vi "CPP-BLplotter.vi"(0 "Plot Array":cluster{dbl[], dbl[]}[](array[cluster]) {"?" format="%.2f"; "?" format="%.2f"}, 1 "Job Directory":path) -> (2 "Saved Automatically?":bool, 3 "gnuplotScript":string, 4 "Plot data file":path)   [LabVIEW 2015]
uses:
  gnuplotScriptComponents/BLPlottersubVIs/BLTarget.ctl
  gnuplotScriptComponents/BLPlottersubVIs/Resampler.ctl
  gnuplotScriptComponents/at.ctl
  Results_plotter_Global.vi
panel:
  in  "Tab Control":enum32{"Good Shit", "Targets", "Boring Shit"}(tab)
  in  "NormaliseHeight?":bool
  in  "oneshot":bool=TRUE
  in  "U(h)":dbl min=0.0 step=0.5
  in  "Fit Zmin":dbl=100.0 min=0.0 max=200.0 step=20.0
  in  "autoprint":bool
  out "with d0":cluster{"n":dbl, "d0":dbl, "d0 2":dbl} {"d0 2" format="%#.1e"; "d0" format="%#.1f"; "n" format="%.3f"}
  in  "Fit Zmax":dbl=550.0 min=0.0 max=2000.0 step=50.0
  out "lambda-":dbl format="%_2g"
  out "lambda+":dbl format="%_2g"
  out "lambda(h)":dbl format="%.3g"
  in  "HeightJitter%":dbl min=0.0 max=20.0 step=1.0
  in  "Spectra Folder::":path
  out "Spectrum":cluster{"all rows":dbl[], "all rows":dbl[]}[](graph)
  in  "Stop Button":bool
  in  "Print Button":bool
  out "U,L(U)":cluster{dbl[], dbl[]}[](graph)
  out "TI,Sigma":cluster{dbl[], dbl[]}[](graph)
  in  "MaxFitFreq":dbl
  in  "lambdaSpan(%)":dbl
  in  "integralTweak":dbl=1.0 min=0.8 max=3.0 step=0.01
  out "case":string
  out "No d0":cluster{"n":dbl, "d0":dbl, "d0 2":dbl} {"d0 2" format="%#.1e"; "n" format="%.3f"}
  in  "Spectra?":bool
  in  "Scale":dbl=1.0 min=1.0 max=10000.0 step=50.0
  in  "Zref":dbl=508.0 min=0.0 step=25.0
  in  "BL Scratchpad":T1[](array[typedef]) {"n" min=0.02 max=0.5 step=0.01 format="%.2f"}
  in  "Boundary Layer Targets Folder":path=path "Data plotting/BLplotterExampleProfiles"
  out "BL Targets":T1[](array[typedef]) {"n" min=0.02 max=0.5 step=0.01 format="%.2f"}
  in  "ScaleInTitle?":bool
  in  "OutputType":enum16{"PDF", "PNG-ReportStyle"}(ring)
  out "File Path Control":path
  in  "Resampler":T2
  in  "ResampleToN":i32=12
  in  "ResampleHeights":dbl[](array[numeric])=[25.4, 38.1, 50.8, 76.2, 101.6, 127.0, 152.4, 203.2, 254.0, 304.8, 406.4, 508.0, 609.6, 812.8, 1219.2, 1524.0]
  in  "Use for:":T3(array[ring])=[enum."\nU", enum."\nLambda", enum."\nTI", enum."\nSigma"]
  out "Incoming Titles":string[](array[string])
  in  "Plot Title":u16(ring) items=["Title String Only", "X:Ref:", "Z:Ref:", "Uref::", "X::", "Y::", "Z::", "U/U_{ref}::", "TI(U)::(%)", "\\lambda(U)::(mm)", "\\sigma(U)/U_{ref}::", "U::", "Var(U)::", "tau(U)::", "Spire::", "Trip::", "Rough::", "Addl::", "Date::", "Seconds::", "Comments::", "Run:Messages:", "Reference:Temperature:Used for Corrections", "Atmos:Pressure:Used for Corrections", "Multi Run:Start Time:", "Measuring:Instrument:Type", "Descpn::", "Multi Run:Row:Type", "Raw:Data:Filename", "Original:Results:Filename", "Current:Data:Filename", "Source::", "n:Regular: Z 80.0 - 800.0", "nd:Regular: Z 80.0 - 800.0", "d0:Regular: Z 80.0 - 800.0", "TI:at:200", "TI:at:400", "TI:at:800", "CandidateFor::", "Z-d::", "Trip:Loc:", "Spires:Loc:", "Number of Measurements"]
  out "Final Title":string
  in  "Plot Title Post Block":string
  in  "Plot Title Pre Block":string="Test"
  in  "Show Script Editor?":bool
  in  "OpenLogfile?":bool
  out "spectraLegend":string[](array[string])
  in  "SpecificPlotFolder":string="DescriptiveFolderName"
  # "Fit using values at  measurement Z heights"
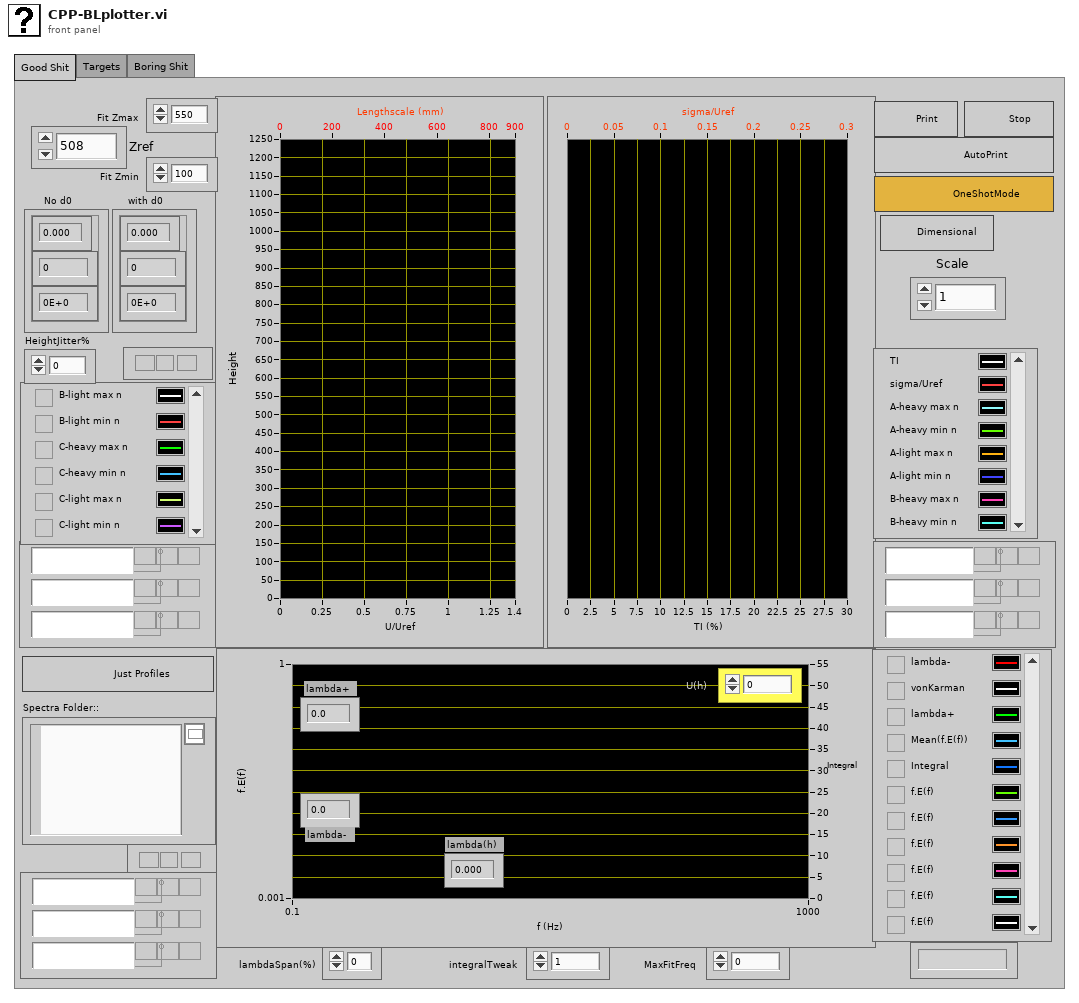
[diagram p1: front panel]
types:
  T1 = typedef "BLTarget.ctl" = cluster{"Code":string, "TI Profile (FS)":dbl[][], "n":dbl}
  T2 = typedef "Resampler.ctl" = enum32{"AsTaken", "Regular", "Prescribed"}
  T3 = enum16{"Don't Use", "\nU", "\nLambda", "\nTI", "\nSigma"}[]
  T4 = typedef "at.ctl" = cluster{"XcoordSys":string, "YcoordSys":string, "Xvalue":dbl, "Yvalue":dbl}
  T5 = typedef "LVRangeTypeDef.ctl" = cluster{"Minimum":dbl, "Maximum":dbl, "Increment":dbl, "Minor Increment":dbl, "Start":dbl}
  T6 = typedef "PowerLaw.ctl" = cluster{"n":dbl, "d0":dbl, "Residual":dbl}
  T7 = cluster{"TI Profile (FS)":dbl[], "Array":dbl[]}[]
  T8 = cluster{"Array":dbl[], "best nonlinear fit":dbl[]}
  T9 = cluster{"Plot.Plot Name":string, "Plot.Plot Color":u32, "Plot.Visible?":bool}
  T10 = typedef "minAndMax.ctl" = cluster{"Min":T11, "Max":T11}
  T11 = typedef "AutoManualNumber.ctl" = cluster{"Auto":bool, "Value":dbl}
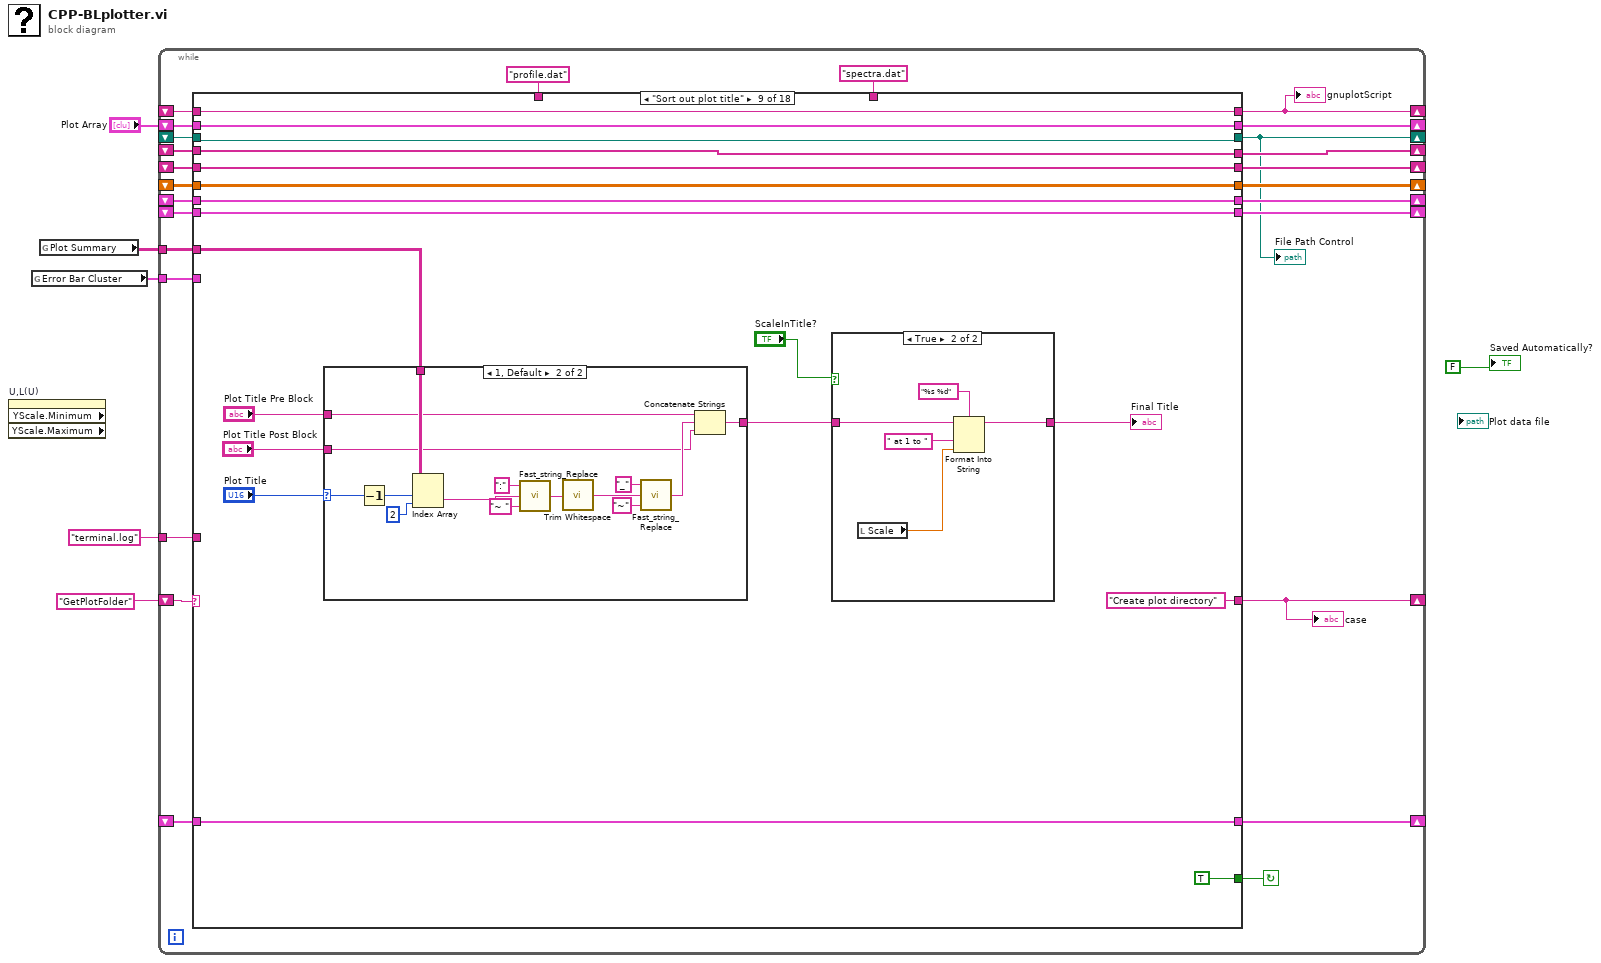
[diagram p0: block diagram]
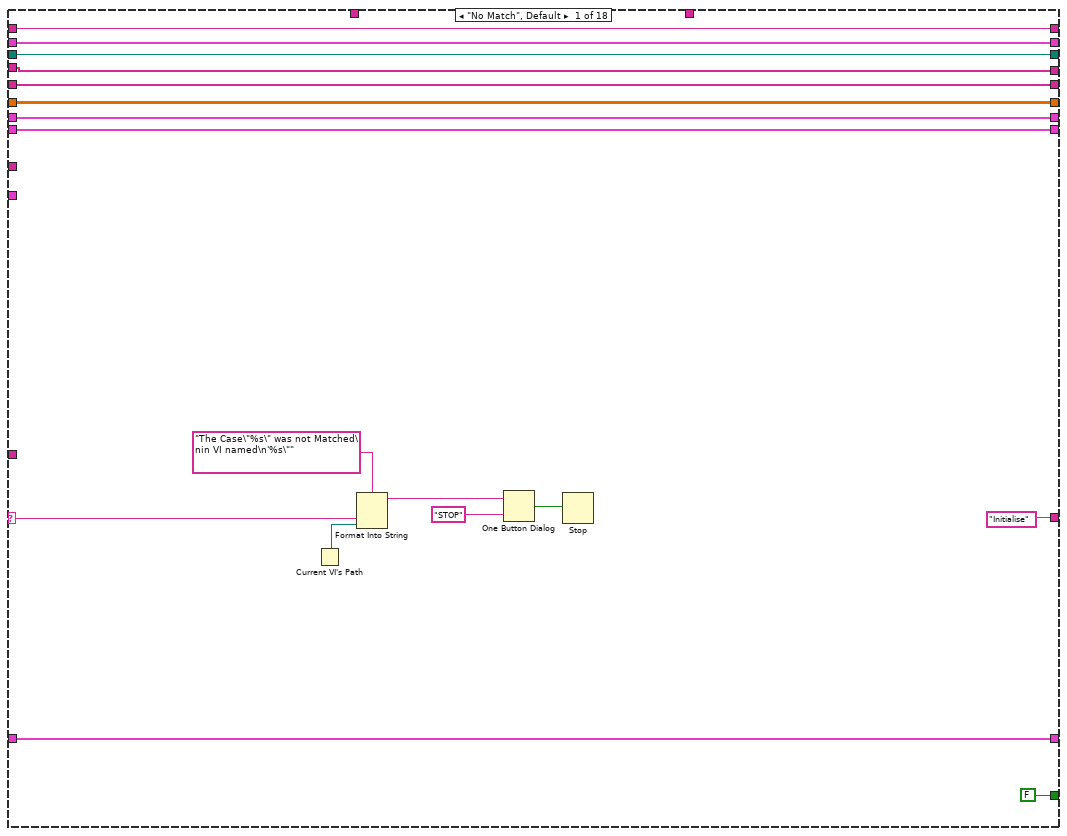
[diagram p2: hidden frame]
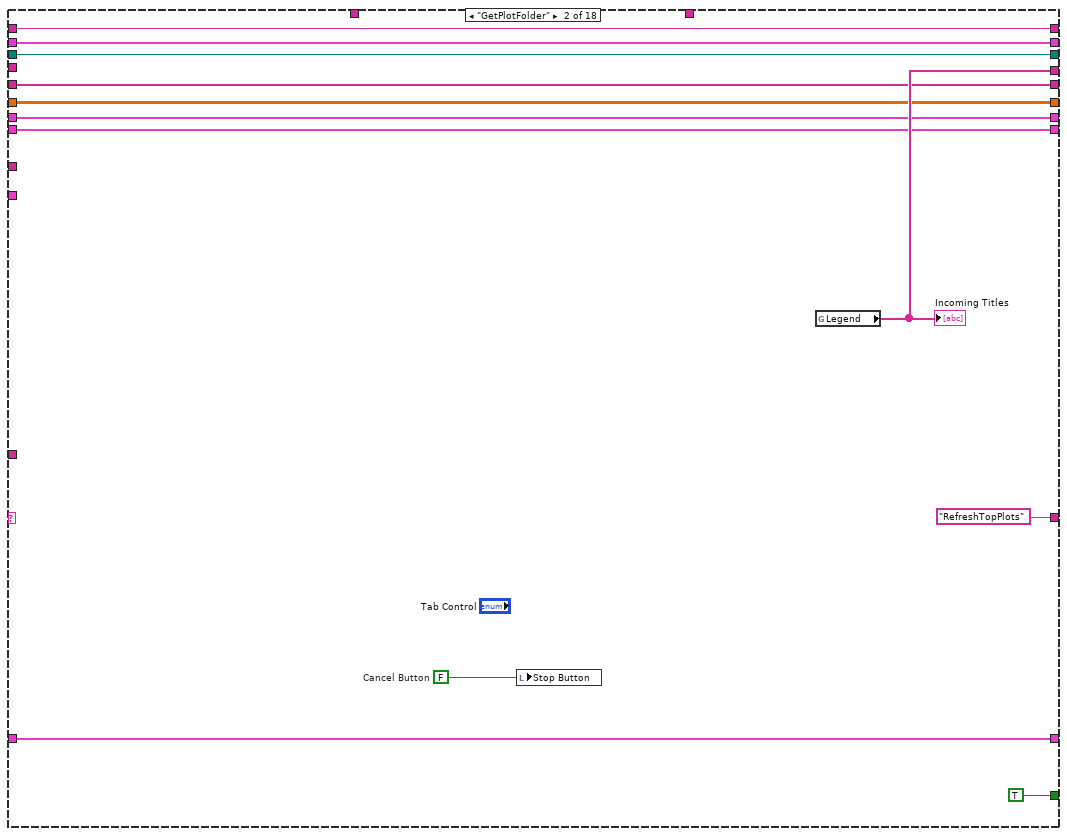
[diagram p3: hidden frame]
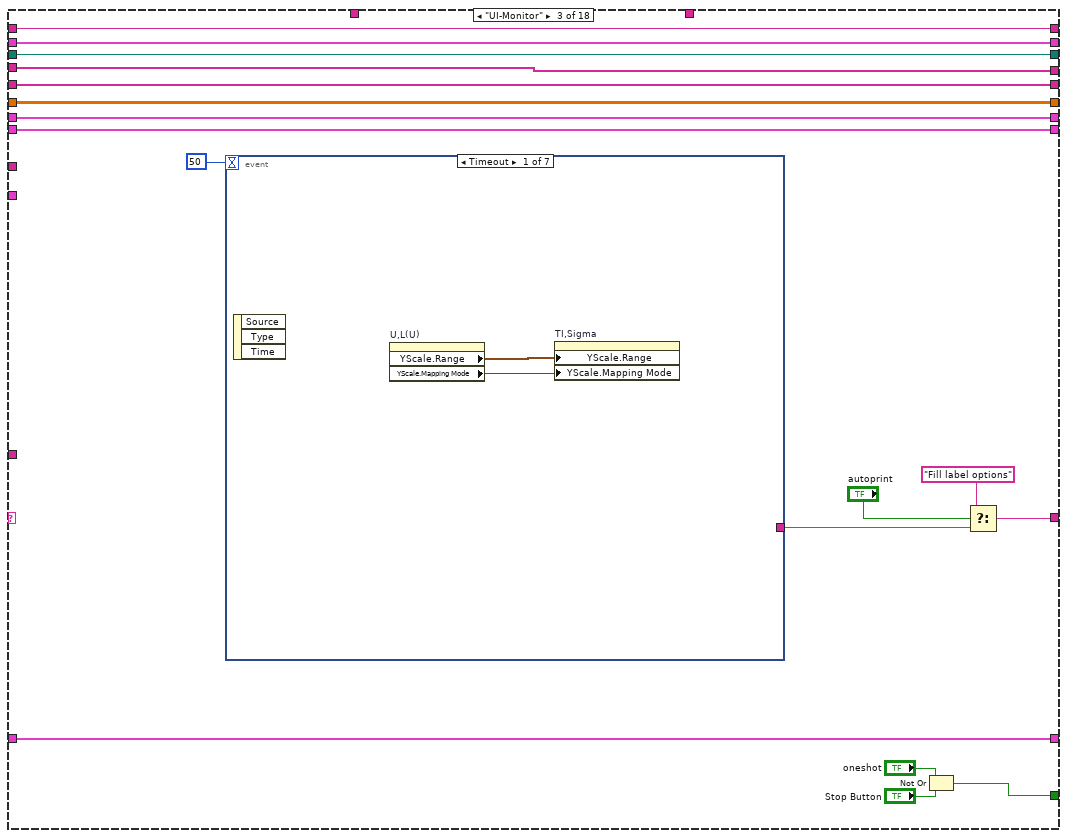
[diagram p4: hidden frame]
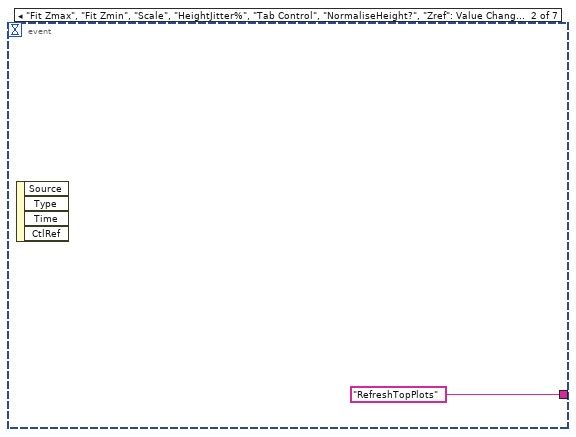
[diagram p5: hidden frame]
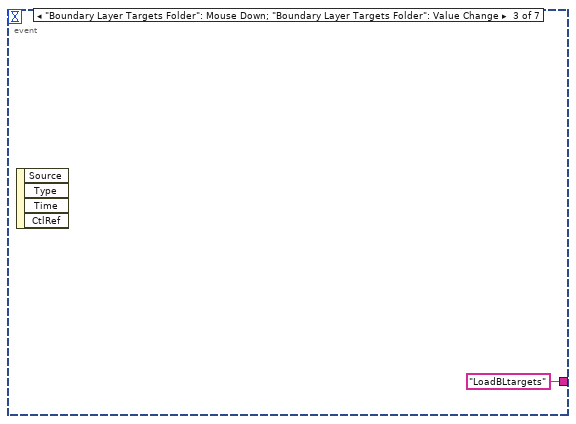
[diagram p6: hidden frame]
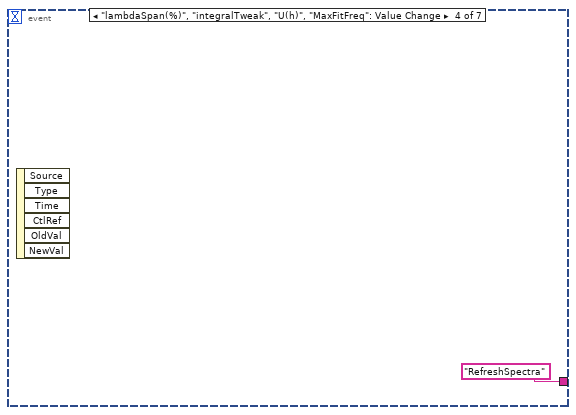
[diagram p7: hidden frame]
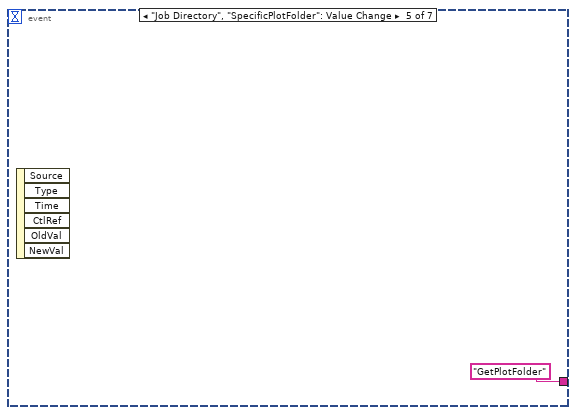
[diagram p8: hidden frame]
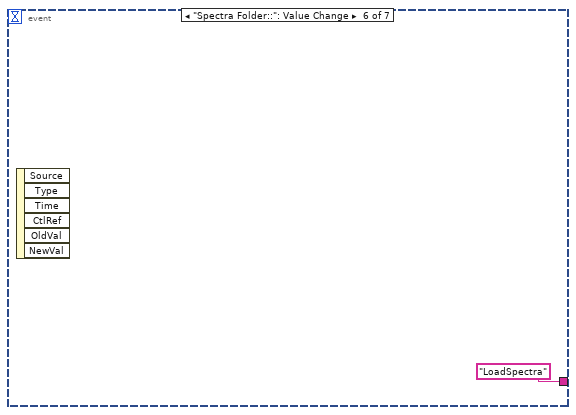
[diagram p9: hidden frame]
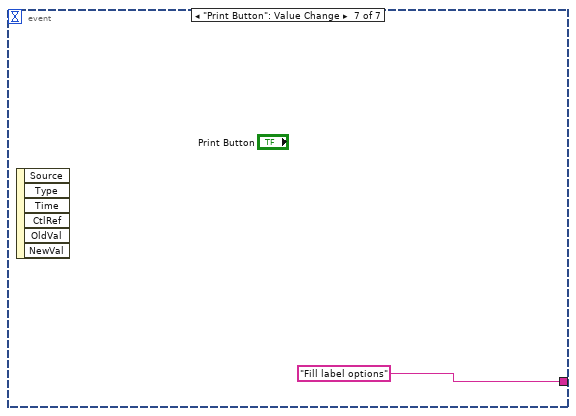
[diagram p10: hidden frame]
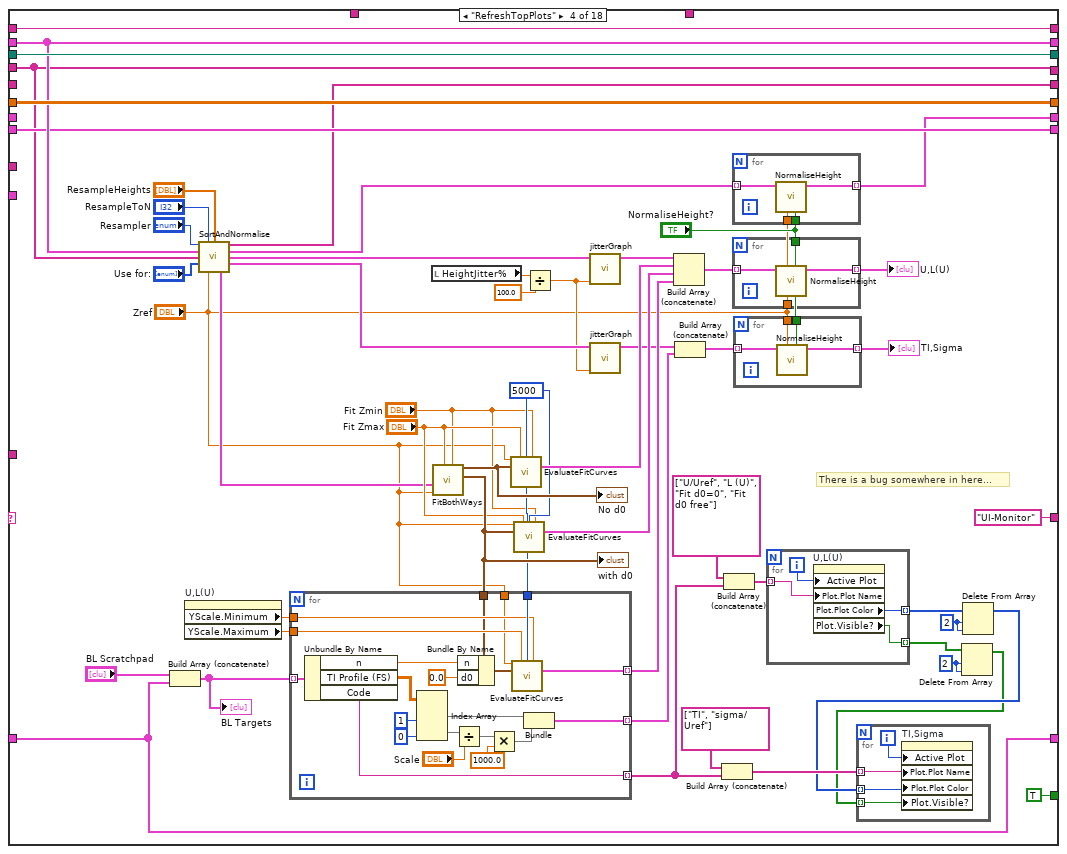
[diagram p11: hidden frame]
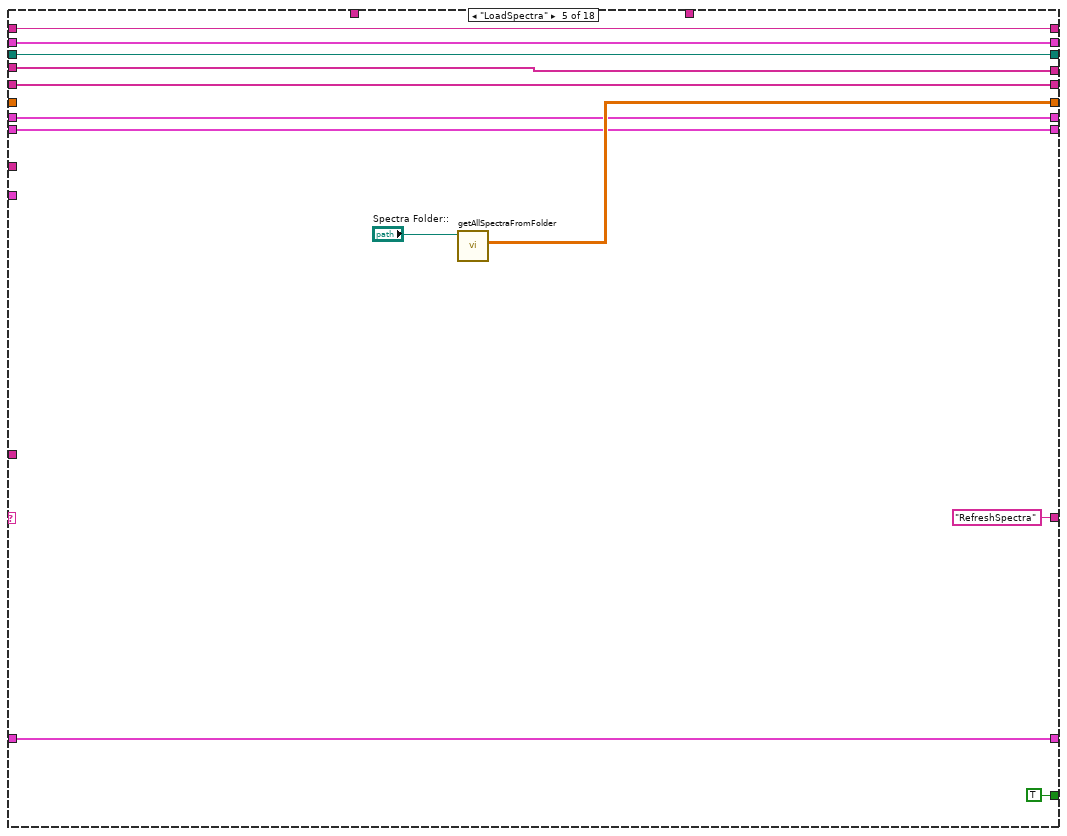
[diagram p12: hidden frame]
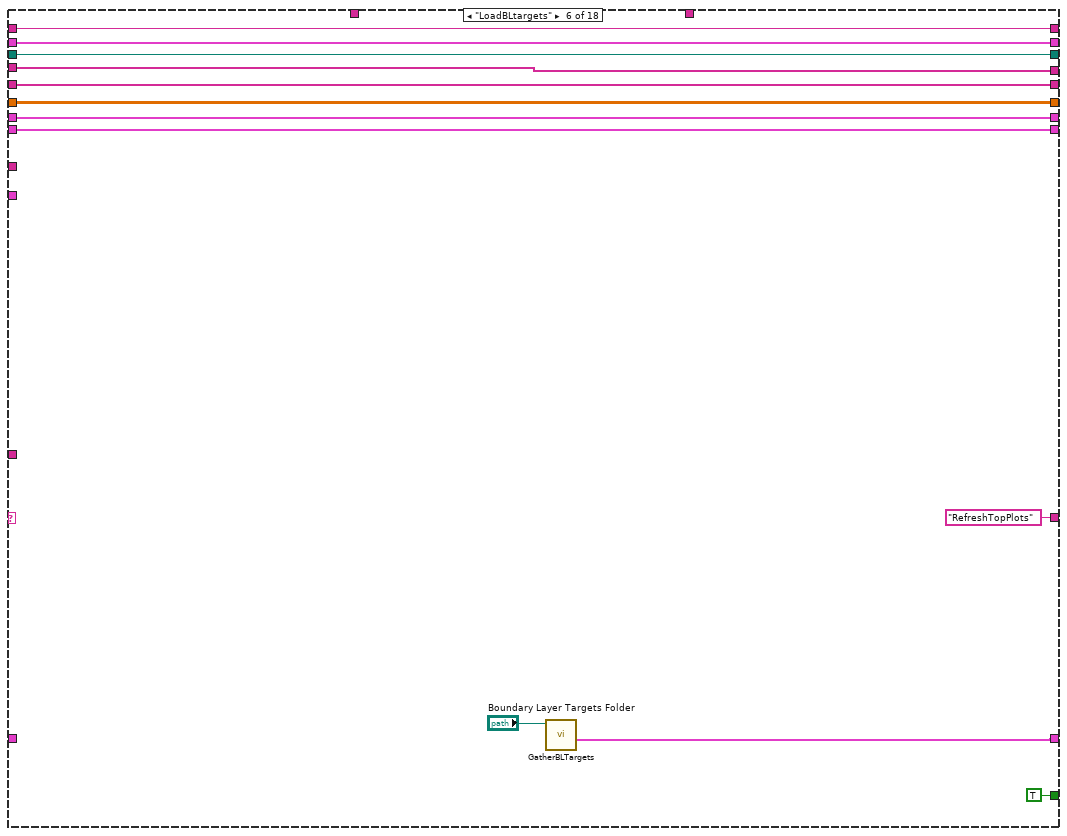
[diagram p13: hidden frame]
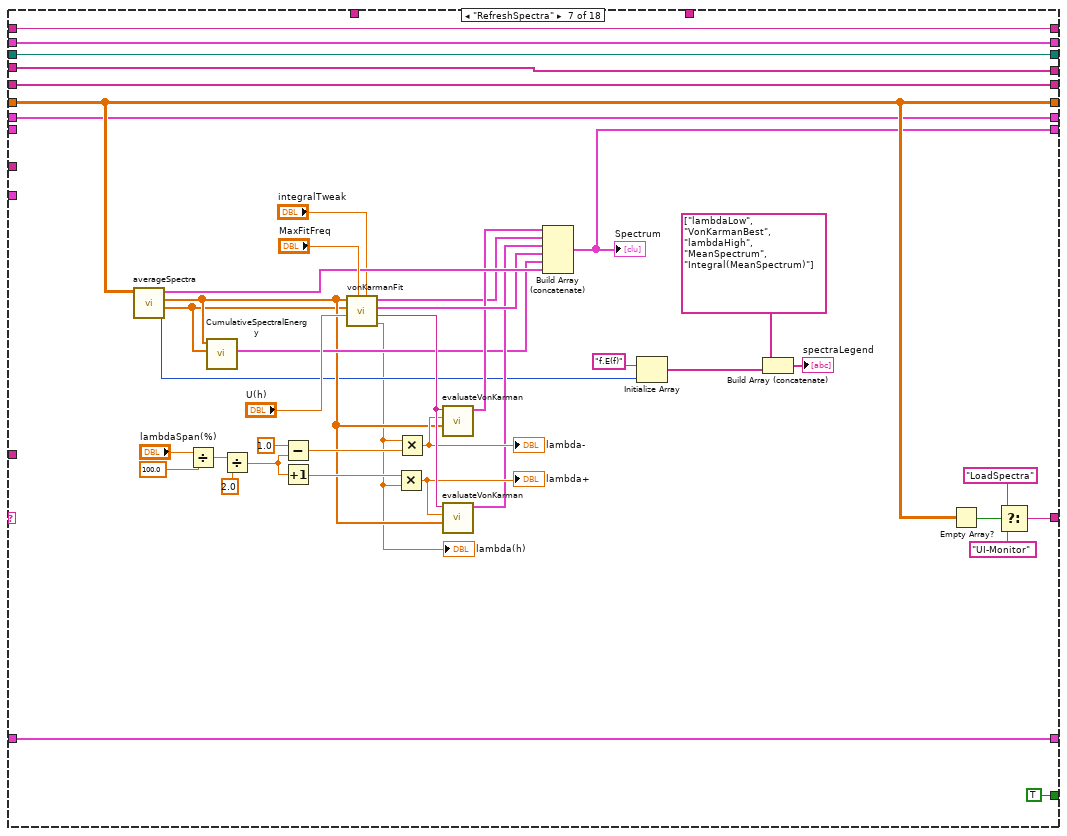
[diagram p14: hidden frame]
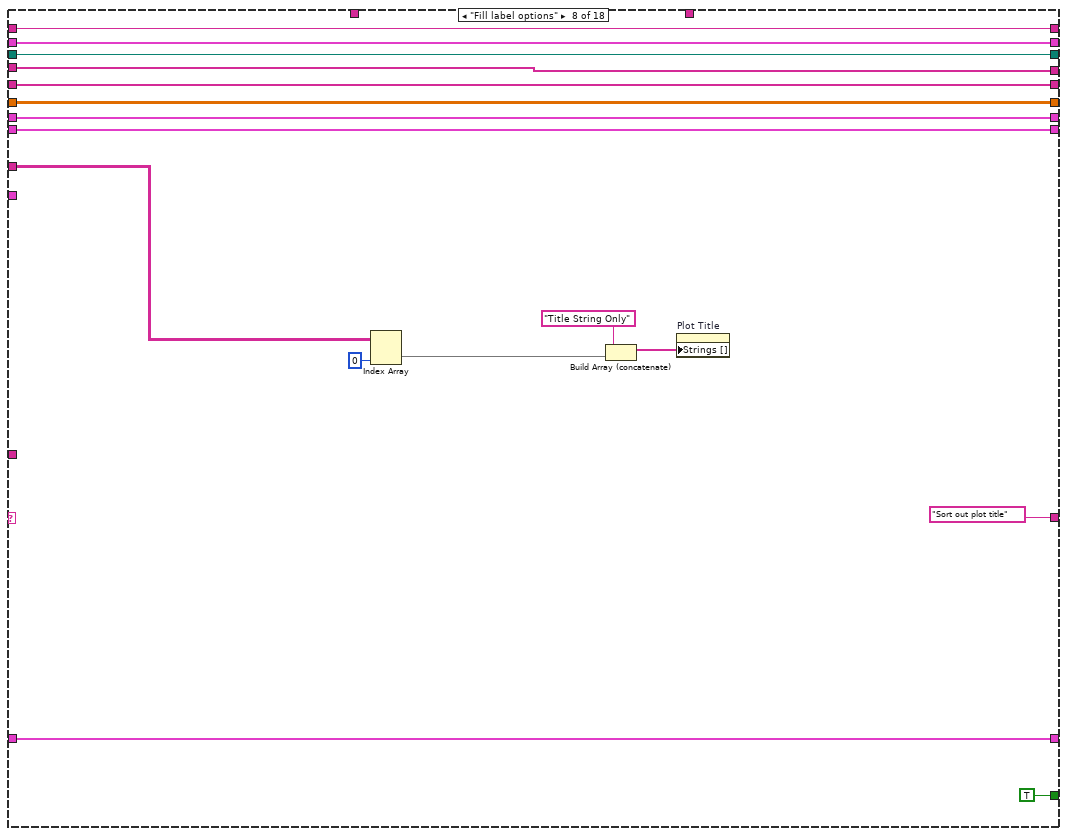
[diagram p15: hidden frame]
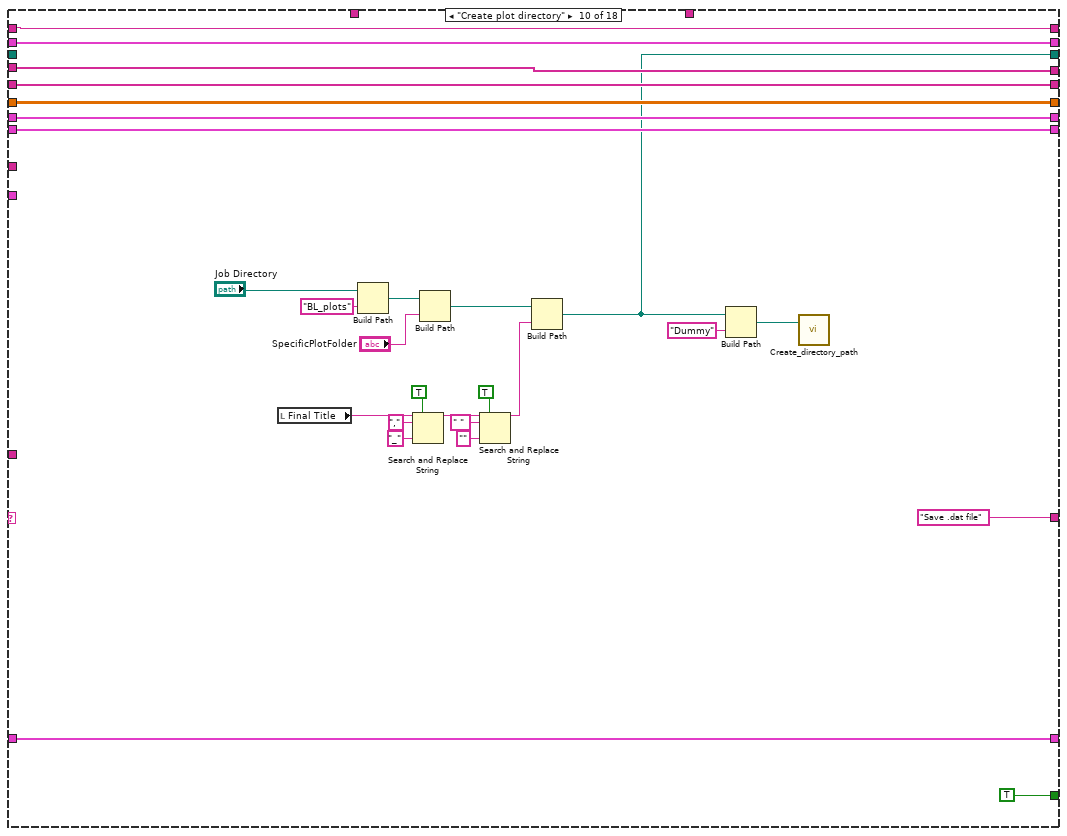
[diagram p18: hidden frame]
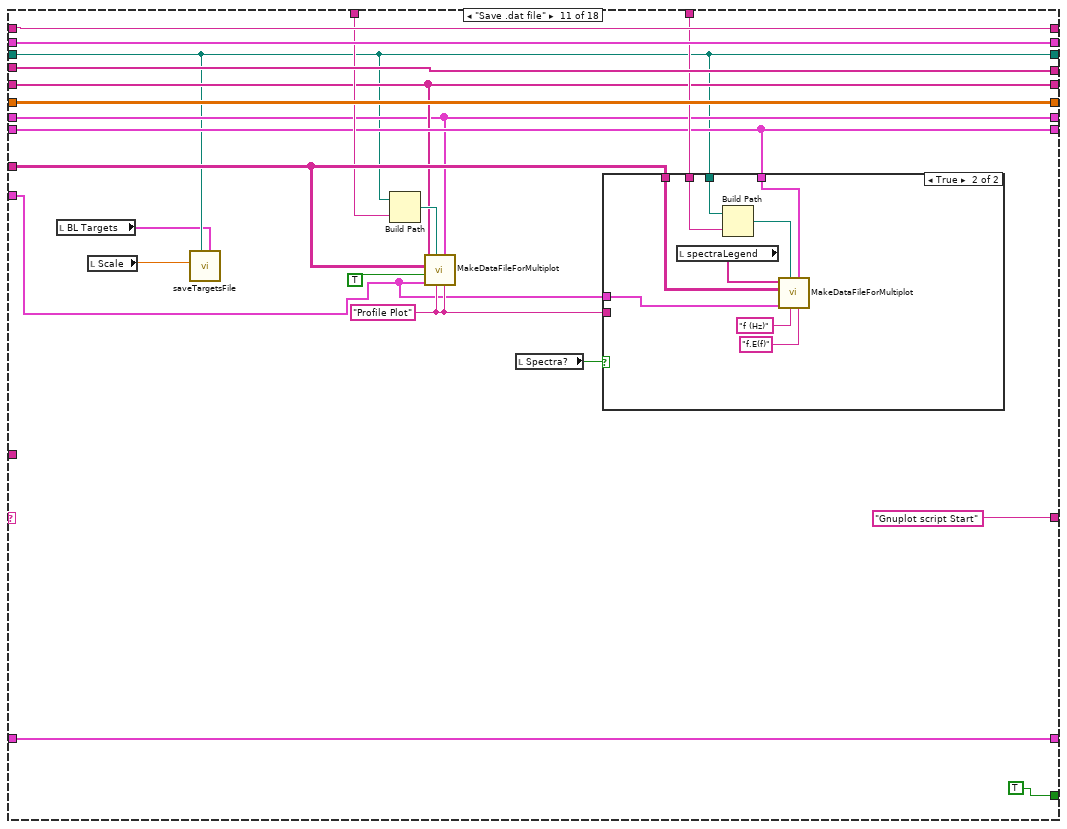
[diagram p19: hidden frame]
diagram:
  n1 = property on="U,L(U)" class="XYGraph (strict)" props=["YScale", "Minimum", "YScale", "Maximum"]() -> ()  [unwired: 2 in, 4 out]
  n2 = global read "Results_plotter_Global.vi" "Error Bar Cluster"() -> (w1:cluster{string[]}[])
  n3 = global read "Results_plotter_Global.vi" "Plot Summary"() -> (w5:string[][])
  n4 = while {
    shift-left: "GetPlotFolder" -> [w31]
    shift-right: [w24] -> _
    tunnel: w5 -> [w30]
    shift-right: [w9] -> _
    shift-left: _ -> [w29]
    shift-right: [w15] -> _
    shift-left: "Plot Array" -> [w28]
    shift-right: [w21] -> _
    shift-left: _ -> [w27]
    shift-right: [w13] -> _
    shift-left: _ -> [w26]
    tunnel: "terminal.log" -> [w25]
    shift-right: [w23] -> _
    shift-left: _ -> [w22]
    shift-right: [w20] -> _
    shift-left: _ -> [w19]
    shift-right: [w16] -> _
    shift-left: _ -> [w14]
    shift-right: [w12] -> _
    shift-left: _ -> [w11]
    tunnel: w1 -> [w10]
    shift-right: [w7] -> _
    shift-left: _ -> [w8]
    stop <- w32 continue-if-true
    n5 = case shown="\"Sort out plot title\"" w31 {
      selector: w31 -> [w38 _ _ _ _ _ _ _ _ _ _ _ _ _ _ _ _ _]
      tunnel: [FALSE TRUE w63 TRUE ("Top Level") TRUE ("Top Level") TRUE ("Top Level") TRUE ("Top Level") TRUE ("Top Level") TRUE ("Top Level") TRUE TRUE ("Top Level") TRUE ("Top Level") TRUE ("Top Level") TRUE ("Top Level") TRUE ("Top Level") w512 TRUE ("Top Level") TRUE ("Top Level")] -> w32
      tunnel: ["Initialise" "RefreshTopPlots" w69 "UI-Monitor" ("t") "RefreshSpectra" ("t") "RefreshTopPlots" ("t") w222 "Sort out plot title" "Create plot directory" ("t") "Save .dat file" "Gnuplot script Start" w386 "Write gnuplot file" ("t") "Execute shell script" ("t") "Has pdf been generated?" ("t") w521 "UI-Monitor" ("t") "UI-Monitor" ("t")] -> w24
      tunnel: w30 -> [_ _ _ _ _ _ _ w264 w277 _ w346 _ _ _ _ _ _ _]
      tunnel: [w42 w51 w75 w141 w194 w206 w248 w259 w272 w320 w337 w391 w472 w480 w496 w524 w533 w543] -> w9
      tunnel: w29 -> [w42 w51 w75 w141 w194 w206 w248 w259 w272 _ w337 w391 w472 w480 w496 w524 w533 w543]
      tunnel: w28 -> [w41 w58 w76 w135 w193 w205 w247 w260 w282 w331 w348 w396 w471 w490 w509 w527 w539 w553]
      tunnel: [w41 w58 w76 w135 w193 w205 w247 w260 w282 w331 w348 w396 w471 w490 w509 w527 w539 w553] -> w15
      tunnel: w27 -> [w40 w59 w77 w140 w192 w204 w246 w261 w278 w330 w352 _ w457 w475 w507 w525 w537 w551]
      tunnel: [w40 w59 w77 w140 w192 w204 w246 w261 w278 w330 w352 w369 w461 w475 w507 w525 w537 w551] -> w21
      tunnel: [w39 w56 w74 w126 w191 w203 w245 w258 w281 w329 w349 w395 w470 w485 w508 w526 w538 w552] -> w13
      tunnel: w26 -> [w39 _ w74 w126 w191 w203 w245 w258 w281 w329 w349 w395 w470 w485 w508 w526 w538 w552]
      tunnel: w25 -> [_ _ _ _ _ _ _ _ _ _ _ _ _ _ w504 _ _ w547]
      tunnel: [w37 w55 w78 w139 w189 w197 w217 w254 w274 w326 w347 w393 w469 w482 w503 w517 w535 w545] -> w23
      tunnel: w22 -> [w37 w55 w78 w139 _ w197 w217 w254 w274 w326 w347 w393 w469 w482 w503 w517 w535 w545]
      tunnel: [w36 w54 w72 w128 w186 w200 w216 w253 w273 w325 w341 w392 w468 w481 w502 w516 w534 w544] -> w20
      tunnel: w19 -> [w36 w54 w72 w128 w186 w200 _ w253 w273 w325 w341 w392 w468 w481 w502 w516 w534 w544]
      tunnel: "profile.dat" ("name or relative path") -> [_ _ _ _ _ _ _ _ _ _ w345 w379 _ _ _ _ _ _]
      tunnel: "spectra.dat" ("name or relative path") -> [_ _ _ _ _ _ _ _ _ _ w344 _ w460 _ _ _ _ _]
      tunnel: [w35 w53 w71 w90 w185 w199 w210 w251 w270 w322 w339 w390 w467 w479 w501 w515 w532 w542] -> w16
      tunnel: w14 -> [w35 w53 w71 _ w185 w199 w210 w251 w270 w322 w339 w390 w467 w479 w501 w515 w532 w542]
      tunnel: [w34 w52 w70 w125 w184 w198 w209 w250 w269 w321 w340 w389 w466 w478 w500 w514 w531 w541] -> w12
      tunnel: w11 -> [w34 w52 w70 _ w184 w198 w209 w250 w269 w321 w340 w389 w466 w478 w500 w514 w531 w541]
      tunnel: w10 -> [_ _ _ _ _ _ _ _ _ _ w334 _ _ _ _ _ _ _]
      tunnel: w8 -> [w33 w50 w62 w97 w183 _ w208 w249 w268 w305 w332 w380 w441 w473 w492 w510 w529 w540]
      tunnel: [w33 w50 w62 w97 w183 w195 w208 w249 w268 w305 w332 w380 w441 w473 w492 w510 w529 w540] -> w7
      frame "No Match", Default {
        n6 = Current VI's Path() -> (path=w44:path)
        n7 = Format Into String(format string="The Case\"%s\" was not Matched\nin VI named\n'%s\"" ("Format String"), w38, w44) -> (resulting string=w47:string)  [unwired: 2 in, 1 out]
        n8 = One Button Dialog(message=w47, button name ("OK")="STOP") -> (true=w45:bool)
        n9 = Stop(stop? (T)=w45) -> ()
      }
      frame "GetPlotFolder" {
        w57 = FALSE  # Cancel Button
        n10 = local write "Stop Button"(w57) -> ()
        n11 = global read "Results_plotter_Global.vi" "Legend"() -> (w56:string[])
        "Incoming Titles" <- w56
      }
      frame "UI-Monitor" {
        n12 = event shown="[0] Timeout" {
          selector: _ -> [_ _ _ _ _ _ _]
          dyn-events: _ -> [_ _ _ _ _ _ _]
          timeout: 50 -> [_ _ _ _ _ _ _]
          tunnel: ["UI-Monitor" "RefreshTopPlots" "LoadBLtargets" "RefreshSpectra" "GetPlotFolder" "LoadSpectra" "Fill label options"] -> w66
          event Timeout {
            n13 = event-data() -> ()  [unwired: 1 in, 3 out]
            n14 = property on="U,L(U)" class="XYGraph (strict)"() -> ("YScale.Range"=w79:T5, "YScale.Mapping Mode"=w80:u8)  [unwired: 2 in, 2 out]
            n15 = property on="TI,Sigma" class="XYGraph (strict)"("YScale.Range"=w79, "YScale.Mapping Mode"=w80) -> ()  [unwired: 2 in, 2 out]
          }
          event "Fit Zmax", "Fit Zmin", "Scale", "HeightJitter%", "Tab Control", "NormaliseHeight?", "Zref": Value Change; "U,L(U)": Plot Attribute Change {
            n16 = event-data() -> ()  [unwired: 1 in, 4 out]
          }
          event "Boundary Layer Targets Folder": Mouse Down; "Boundary Layer Targets Folder": Value Change {
            n17 = event-data() -> ()  [unwired: 1 in, 4 out]
          }
          event "lambdaSpan(%)", "integralTweak", "U(h)", "MaxFitFreq": Value Change {
            n18 = event-data() -> ()  [unwired: 1 in, 6 out]
          }
          event "Job Directory", "SpecificPlotFolder": Value Change {
            n19 = event-data() -> ()  [unwired: 1 in, 6 out]
          }
          event "Spectra Folder::": Value Change {
            n20 = event-data() -> ()  [unwired: 1 in, 6 out]
          }
          event "Print Button": Value Change {
            n21 = event-data() -> ()  [unwired: 1 in, 6 out]
          }
        }
        n22 = Not Or(1:"Stop Button", 2:"oneshot") -> (0:w63:bool)
        n23 = Select(t="Fill label options", s="autoprint", f=w66) -> (s? t:f=w69:string)
      }
      frame "RefreshTopPlots" {
        w105 = 2 ("length")
        w106 = 2 ("length")
        w118 = 5000
        # "There is a bug somewhere in here..."
        n24 = Build Array (concatenate)("BL Scratchpad", w97) -> (w102:T1[])
        "BL Targets" <- w102
        n25 = property on="U,L(U)" class="XYGraph (strict)"() -> ("YScale.Minimum"=w123:dbl, "YScale.Maximum"=w122:dbl)  [unwired: 2 in, 2 out]
        n26 = call "SortAndNormalise.vi"("Resampler"="Resampler", "ResampleToN"="ResampleToN", "ResampleHeights"="ResampleHeights", "Plot Array In"=w135, "LegendsIn"=w126, "Use for:"="Use for:", "Zref"="Zref") -> ("SortedLegends"=w125:string[], "SortedData"=w91:cluster{"Array":dbl[], "Array":dbl[]}[], "LeftGraph"=w132:cluster{"Array":dbl[], "Array":dbl[]}[], "RightGraph"=w130:cluster{"Array":dbl[], "Array":dbl[]}[], "UzClusterOutput"=w96:cluster{"Array":dbl[], "Array":dbl[]})  [unwired: 4 in]
        n27 = local read "HeightJitter%"() -> (w137:dbl)
        n28 = call "FitBothWays.vi"("Fit Zmin"="Fit Zmin", "Fit Zmax"="Fit Zmax", "Zref"="Zref", "zUCluster in"=w96) -> ("PowerLawWithDisplacement"=w120:T6, "PowerLawNoDisplacement"=w121:T6)  [unwired: 6 in]
        "No d0" <- w121
        "with d0" <- w120
        n29 = for {
          tunnel: [w182] -> w119 mode=indexing
          tunnel: w118 -> [w181]
          tunnel: w123 -> [w180]
          tunnel: w122 -> [w179]
          tunnel: w102 -> [w178] mode=indexing
          tunnel: w120 -> [w176]
          tunnel: [w173] -> w115 mode=indexing
          tunnel: [w163] -> w114 mode=indexing
          tunnel: "Zref" -> [w162]
          n30 = Unbundle By Name(w178) -> ("n"=w175:dbl, "TI Profile (FS)"=w164:dbl[][], "Code"=w163:string)
          n31 = Index Array(array=w164, index (col) #1=1 ("disabled index (col)"), index (col) #2=0 ("index (col)")) -> (element #1=w170:dbl[], element #2=w168:dbl[])  [unwired: 2 in]
          n32 = Divide(x=w168, y="Scale") -> (x/y=w169:dbl[])
          n33 = Bundle By Name(cluster=w176, "n"=w175, "d0"=0.0) -> (w177:T6)
          n34 = Multiply(x=w169, y=1000.0) -> (x*y=w166:dbl[])
          n35 = call "EvaluateFitCurves.vi"("Zref"=w162, "Fit Zmax"=w179, "nPoints"=w181, "Fit Zmin"=w180, "PowerLaw"=w177) -> ("PlotCluster"=w182:cluster{"Array":dbl[], "Array":dbl[]})  [unwired: 10 in]
          n36 = Bundle("TI Profile (FS)"=w170, w166) -> (w173:cluster{"TI Profile (FS)":dbl[], dbl[]})  [unwired: 1 in]
        }
        n37 = call "EvaluateFitCurves.vi"("Zref"="Zref", "Fit Zmax"="Fit Zmax", "nPoints"=w118, "Fit Zmin"="Fit Zmin", "PowerLaw"=w121) -> ("PlotCluster"=w127:cluster{"Array":dbl[], "Array":dbl[]})  [unwired: 10 in]
        n38 = call "EvaluateFitCurves.vi"("Zref"="Zref", "Fit Zmax"="Fit Zmax", "nPoints"=w118, "Fit Zmin"="Fit Zmin", "PowerLaw"=w120) -> ("PlotCluster"=w124:cluster{"Array":dbl[], "Array":dbl[]})  [unwired: 10 in]
        n39 = Divide(x=w137, y=100.0) -> (x/y=w129:dbl)
        n40 = call "jitterGraph.vi"("Y-jitter"=w129, "GraphPlots"=w132) -> ("jitteredGraphPlots"=w131:cluster{"Array":dbl[], "Array":dbl[]}[])  [unwired: 9 in]
        n41 = call "jitterGraph.vi"("Y-jitter"=w129, "GraphPlots"=w130) -> ("jitteredGraphPlots"=w116:cluster{"Array":dbl[], "Array":dbl[]}[])  [unwired: 9 in]
        n42 = Build Array (concatenate)(w131, w127, w124, w119) -> (w95:cluster{"Array":dbl[], "Array":dbl[]}[])
        n43 = Build Array (concatenate)(w116, w115) -> (w93:T7)
        n44 = Build Array (concatenate)(string[] ["TI", "sigma/Uref"], w114) -> (w117:string[])
        n45 = Build Array (concatenate)(string[] ["U/Uref", "L (U)", "Fit d0=0", "Fit d0 free"], w114) -> (w109:string[])
        n46 = for {
          tunnel: w91 -> [w145] mode=indexing
          tunnel: [w144] -> w90 mode=indexing
          tunnel: "Zref" -> [w143]
          tunnel: "NormaliseHeight?" -> [w142]
          n47 = call "NormaliseHeight.vi"("NormaliseHeight?"=w142, "Zref"=w143, "Value-Z Cluster In"=w145) -> ("Value-Z Cluster Out"=w144:cluster{"Array":dbl[], "Array":dbl[]})  [unwired: 8 in]
        }
        n48 = for {
          tunnel: w95 -> [w153] mode=indexing
          tunnel: [w152] -> w94 mode=indexing
          tunnel: "NormaliseHeight?" -> [w151]
          tunnel: "Zref" -> [w150]
          n49 = call "NormaliseHeight.vi"("NormaliseHeight?"=w151, "Zref"=w150, "Value-Z Cluster In"=w153) -> ("Value-Z Cluster Out"=w152:cluster{"Array":dbl[], "Array":dbl[]})  [unwired: 8 in]
        }
        "U,L(U)" <- w94
        n50 = for {
          tunnel: w93 -> [w149] mode=indexing
          tunnel: [w148] -> w92 mode=indexing
          tunnel: "NormaliseHeight?" -> [w147]
          tunnel: "Zref" -> [w146]
          n51 = call "NormaliseHeight.vi"("NormaliseHeight?"=w147, "Zref"=w146, "Value-Z Cluster In"=w149) -> ("Value-Z Cluster Out"=w148:cluster{"Array":dbl[], "Array":dbl[]})  [unwired: 8 in]
        }
        "TI,Sigma" <- w92
        n52 = for {
          tunnel: w109 -> [w158] mode=indexing
          tunnel: [w161] -> w108 mode=indexing
          tunnel: [w160] -> w104 mode=indexing
          i -> [w159]
          n53 = property on="U,L(U)" class="XYGraph (strict)"("Active Plot"=w159, "Plot.Plot Name"=w158) -> ("Plot.Plot Color"=w161:u32, "Plot.Visible?"=w160:bool)  [unwired: 2 in, 2 out]
        }
        n54 = Delete From Array(array=w104, length=w105, index=w105) -> (array with subset deleted=w103:bool[])  [unwired: 1 out]
        n55 = Delete From Array(array=w108, length=w106, index=w106) -> (array with subset deleted=w107:u32[])  [unwired: 1 out]
        n56 = for {
          tunnel: w117 -> [w154] mode=indexing
          tunnel: w107 -> [w157] mode=indexing
          tunnel: w103 -> [w156] mode=indexing
          i -> [w155]
          n57 = property on="TI,Sigma" class="XYGraph (strict)"("Active Plot"=w155, "Plot.Plot Name"=w154, "Plot.Plot Color"=w157, "Plot.Visible?"=w156) -> ()  [unwired: 2 in, 2 out]
        }
      }
      frame "LoadSpectra" {
        n58 = call "getAllSpectraFromFolder.vi"("Spectra Folder::"="Spectra Folder::") -> ("spectra"=w189:dbl[][][])  [unwired: 10 in]
      }
      frame "LoadBLtargets" {
        n59 = call "GatherBLTargets.vi"("BL files folder path"="Boundary Layer Targets Folder") -> ("BL Targets out"=w195:T1[])  [unwired: 10 in]
      }
      frame "RefreshSpectra" {
        n60 = call "averageSpectra.vi"("multipleSpectra"=w217) -> ("nSpectra"=w214:i32, "meanSpectrum"=w218:dbl[], "frequencies"=w219:dbl[], "spectraPlots"=w242:cluster{"Array":dbl[], "Array":dbl[]}[])  [unwired: 7 in]
        n61 = Divide(x="lambdaSpan(%)", y=100.0) -> (x/y=w235:dbl)
        n62 = call "CumulativeSpectralEnergy.vi"("f.E(f)"=w218, "f"=w219) -> ("plottableBundle"=w226:cluster{"X":dbl[], "Array":dbl[]})  [unwired: 8 in, 1 out]
        n63 = Divide(x=w235, y=2.0 ("x")) -> (x/y=w228:dbl)
        n64 = Subtract(x=1.0, y=w228) -> (x-y=w237:dbl)
        n65 = Increment(x=w228) -> (x+1=w236:dbl)
        n66 = call "vonKarmanFit.vi"("integralTweak"="integralTweak", "MaxFitFreq"="MaxFitFreq", "U(h)"="U(h)", "f.E(f)"=w218, "f"=w219) -> ("lambda"=w207:dbl, "vonKarmanFitEquation"=w240:string, "CroppedData"=w241:cluster{"X Out":dbl[], "Y Out":dbl[]}, "FitCurve"=w230:T8)  [unwired: 3 in]
        "lambda(h)" <- w207
        n67 = Multiply(x=w236, y=w207) -> (x*y=w231:dbl)
        "lambda+" <- w231
        n68 = Multiply(x=w207, y=w237) -> (x*y=w232:dbl)
        "lambda-" <- w232
        n69 = call "evaluateVonKarman.vi"("frequencies"=w219, "lambda"=w232, "vonKarmanFitEquation"=w240) -> ("Cluster"=w233:cluster{"frequencies":dbl[], "Y Values":dbl[]})  [unwired: 8 in]
        n70 = call "evaluateVonKarman.vi"("frequencies"=w219, "lambda"=w231, "vonKarmanFitEquation"=w240) -> ("Cluster"=w229:cluster{"frequencies":dbl[], "Y Values":dbl[]})  [unwired: 8 in]
        n71 = Build Array (concatenate)(w233, w230, w229, w241, w226, w242) -> (w216:cluster{"Array":dbl[], "Array":dbl[]}[])
        "Spectrum" <- w216
        n72 = Initialize Array("f.E(f)", w214) -> (w213:string[])
        n73 = Build Array (concatenate)(string[] ["lambdaLow", "VonKarmanBest", "lambdaHigh", "MeanSpectrum", "Integral(MeanSpectrum)"], w213) -> (→"spectraLegend":string[])
        n74 = Empty Array?(array=w217) -> (empty?=w221:bool)
        n75 = Select(t="LoadSpectra", s=w221, f="UI-Monitor" ("t")) -> (s? t:f=w222:string)
      }
      frame "Fill label options" {
        n76 = Index Array(array=w264, index (col)=0 ("disabled index (col)")) -> (element=w256:string[])  [unwired: 1 in]
        n77 = Build Array (concatenate)("Title String Only", w256) -> (w255:string[])
        n78 = property on="Plot Title" class="Ring (strict)"("Strings []"=w255) -> ()  [unwired: 2 in, 2 out]
      }
      frame "Sort out plot title" {
        n79 = case shown="1, Default" "Plot Title" {
          selector: "Plot Title" -> [_ w290]
          tunnel: [w289 w295] -> w267
          tunnel: "Plot Title Pre Block" -> [w289 w294]
          tunnel: w277 -> [_ w297]
          tunnel: "Plot Title Post Block" -> [_ w291]
          frame 0 {
          }
          frame 1, Default {
            n80 = Decrement(x=w290) -> (x-1=w296:u16)
            n81 = Index Array(array=w297, index (row)=w296, index (col)=u16 2 ("y")) -> (element=w300:string)
            n82 = call "Fast_string_Replace.vi"("Replace match with:"="~ ", "Input String"=w300, "regular expression"=":") -> ("Output String"=w299:string)  [unwired: 2 out]
            n83 = call <vilib>:"Trim Whitespace.vi"("string"=w299) -> ("trimmed string"=w298:string)  [unwired: 1 in]
            n84 = call "Fast_string_Replace.vi"("Replace match with:"="~", "Input String"=w298, "regular expression"="_") -> ("Output String"=w293:string)  [unwired: 2 out]
            n85 = Concatenate Strings(w294, w293, w291) -> (w295:string)
          }
        }
        n86 = case shown="True" "ScaleInTitle?" {
          tunnel: w267 -> [w283 w288]
          tunnel: [w283 w284] -> w266
          frame False {
          }
          frame True {
            n87 = local read "Scale"() -> (w287:dbl)
            n88 = Format Into String(format string="%s %d", initial string=w288, " at 1 to " ("string"), w287) -> (resulting string=w284:string)  [unwired: 1 in, 1 out]
          }
        }
        "Final Title" <- w266
      }
      frame "Create plot directory" {
        n89 = local read "Final Title"() -> (w319:string)
        n90 = Build Path(base path="Job Directory", name or relative path="BL_plots") -> (appended path=w306:path)
        n91 = Search and Replace String(replace all?=TRUE ("replace all? (F)"), input string=w319, search string=",", replace string="_" ("replace string (\"\")")) -> (result string=w312:string)  [unwired: 4 in, 3 out]
        n92 = Build Path(base path=w306, name or relative path="SpecificPlotFolder") -> (appended path=w309:path)
        n93 = Search and Replace String(replace all?=TRUE ("replace all? (F)"), input string=w312, search string=" ", replace string="" ("replace string (\"\")")) -> (result string=w311:string)  [unwired: 4 in, 3 out]
        n94 = Build Path(base path=w309, name or relative path=w311) -> (appended path=w320:path)
        n95 = Build Path(base path=w320, name or relative path="Dummy") -> (appended path=w324:path)
        n96 = call "Create_directory_path.vi"("Path name"=w324) -> ()  [unwired: 1 in, 2 out]
      }
      frame "Save .dat file" {
        w338 = "Profile Plot" ("X Axis Name")
        n97 = local read "BL Targets"() -> (w336:T1[])
        n98 = local read "Scale"() -> (w335:dbl)
        n99 = call "saveTargetsFile.vi"("BL Targets"=w336, "Path"=w337, "Scale"=w335) -> ()  [unwired: 9 in]
        n100 = Build Path(base path=w337, name or relative path=w345) -> (appended path=w342:path)
        n101 = call "MakeDataFileForMultiplot.vi"("Y Axis Name"=w338, "Plot Array"=w339, "X Axis Name"=w338, "Path"=w342, "Error Bar Cluster"=w334, "Transpose"=TRUE, "Plot Summary"=w346, "Legend"=w340) -> ()  [unwired: 4 in]
        n102 = local read "Spectra?"() -> (w333:bool)
        n103 = case shown="True" w333 {
          tunnel: w346 -> [_ w361]
          tunnel: w344 -> [_ w360]
          tunnel: w341 -> [_ w359]
          tunnel: w338 -> [_ _]
          tunnel: w337 -> [_ w358]
          tunnel: w334 -> [_ w357]
          frame False {
          }
          frame True {
            n104 = local read "spectraLegend"() -> (w353:string[])
            n105 = Build Path(base path=w358, name or relative path=w360) -> (appended path=w354:path)
            n106 = call "MakeDataFileForMultiplot.vi"("Y Axis Name"="f.E(f)", "Plot Array"=w359, "X Axis Name"="f (Hz)", "Path"=w354, "Error Bar Cluster"=w357, "Plot Summary"=w361, "Legend"=w353) -> ()  [unwired: 5 in]
          }
        }
      }
      frame "Gnuplot script Start" {
        # "Number of \"permanent\" plots"
        # "Number of \"permanent\" plots"
        n107 = local read "BL Targets"() -> (w365:T1[])
        n108 = Array Size(array=w365) -> (size(s)=w381:i32)
        n109 = Add(x=w381, y=4 ("x")) -> (x+y=w384:i32)
        n110 = for {
          N: w384 -> [_]
          tunnel: [w437] -> w364 mode=indexing
          i -> [w436]
          n111 = property on="U,L(U)" class="XYGraph (strict)"("Active Plot"=w436) -> ("Plot.Plot Name"=w440:string, "Plot.Plot Color"=w439:u32, "Plot.Visible?"=w438:bool)  [unwired: 2 in, 2 out]
          n112 = Bundle("Plot.Plot Name"=w440, "Plot.Plot Color"=w439, "Plot.Visible?"=w438) -> (w437:T9)  [unwired: 1 in]
        }
        n113 = local read "NormaliseHeight?"() -> (w376:bool)
        n114 = Add(x=w381, y=2 ("x")) -> (x+y=w382:i32)
        n115 = for {
          N: w382 -> [_]
          tunnel: [w433] -> w363 mode=indexing
          i -> [w431]
          n116 = property on="TI,Sigma" class="XYGraph (strict)"("Active Plot"=w431) -> ("Plot.Plot Name"=w432:string, "Plot.Plot Color"=w435:u32, "Plot.Visible?"=w434:bool)  [unwired: 2 in, 2 out]
          n117 = Bundle("Plot.Plot Name"=w432, "Plot.Plot Color"=w435, "Plot.Visible?"=w434) -> (w433:T9)  [unwired: 1 in]
        }
        n118 = local read "Final Title"() -> (w378:string)
        n119 = local read "Fit Zmax"() -> (w374:dbl)
        n120 = control-ref of="TI,Sigma"() -> (w366:refnum<vi>)
        n121 = control-ref of="U,L(U)"() -> (w367:refnum<vi>)
        n122 = local read "Fit Zmin"() -> (w373:dbl)
        n123 = local read "with d0"() -> (w370:cluster{"n":dbl, "d0":dbl, "d0 2":dbl})
        n124 = local read "No d0"() -> (w371:cluster{"n":dbl, "d0":dbl, "d0 2":dbl})
        n125 = local read "Scale"() -> (w368:dbl)
        n126 = local read "Zref"() -> (w375:dbl)
        n127 = case shown="\"PDF\", Default" "OutputType" {
          tunnel: w379 -> [w413 w430]
          tunnel: w378 -> [w412 w429]
          tunnel: "Spectra?" -> [w411 w428]
          tunnel: w376 -> [w410 w427]
          tunnel: w375 -> [w409 w426]
          tunnel: w374 -> [w408 w425]
          tunnel: w373 -> [w407 w424]
          tunnel: "HeightJitter%" -> [w406 w423]
          tunnel: w371 -> [w405 w422]
          tunnel: w370 -> [w404 w421]
          tunnel: [w403 w420] -> w369
          tunnel: w368 -> [w402 w419]
          tunnel: w367 -> [w401 w418]
          tunnel: w366 -> [w400 w417]
          tunnel: w365 -> [w399 w416]
          tunnel: w364 -> [w398 w415]
          tunnel: w363 -> [w397 w414]
          frame "PDF", Default {
            n128 = call "AssembleBLMultiplotScript-UandTI.vi"("name or relative path"=w413, "Final Title"=w412, "Spectra?"=w411, "NormaliseHeight?"=w410, "Zref"=w409, "Fit Zmax"=w408, "Fit Zmin"=w407, "HeightJitter%"=w406, "Scale"=w402, "BL Targets"=w399, "U,L(U)"=w401, "UtargetsInfo"=w398, "TI,Sigma"=w400, "TItargetsInfo"=w397, "No d0"=w405, "with d0"=w404) -> ("gnuplotOut"=w403:string)  [unwired: 11 in]
          }
          frame "PNG-ReportStyle" {
            n129 = call "AssembleBLMultiplotScript-UandTI-CPPPNG.vi"("name or relative path"=w430, "Final Title"=w429, "Spectra?"=w428, "NormaliseHeight?"=w427, "Zref"=w426, "Fit Zmax"=w425, "Fit Zmin"=w424, "HeightJitter%"=w423, "Scale"=w419, "BL Targets"=w416, "U,L(U)"=w418, "UtargetsInfo"=w415, "TI,Sigma"=w417, "TItargetsInfo"=w414, "No d0"=w422, "with d0"=w421) -> ("gnuplotOut"=w420:string)  [unwired: 11 in]
          }
        }
        n130 = Select(t="spectraScript", s="Spectra?", f="Write gnuplot file" ("t")) -> (s? t:f=w386:string)
      }
      frame "spectraScript" {
        w455 = 1.0 ("Width")
        w456 = 0.0 ("LateralPosition")
        w462 = 0 ("Active Y Scale")
        n131 = local read "lambda(h)"() -> (w450:dbl)
        n132 = local read "U(h)"() -> (w446:dbl)
        n133 = call "SetSizeAndOriginForMultiplot.vi"("VerticalPosition"=w456, "Height"=w455, "LateralPosition"=w456, "Width"=w455, "ClearLabels?"=TRUE, "PlotLocationDescription"="Bottom plot", "gnuplotIn"=w457) -> ("gnuplotOut"=w452:string)  [unwired: 4 in]
        n134 = Format Into String(format string="$\\\\lambda= %0.2f$m", w450) -> (resulting string=w443:string)  [unwired: 2 in, 1 out]
        n135 = Format Into String(format string="$U(h)= %0.2f$ms$^{-1}$", w446) -> (resulting string=w444:string)  [unwired: 2 in, 1 out]
        n136 = Build Array(w444, w443) -> (w442:string[])
        n137 = control-ref of="Spectrum"() -> (w465:refnum<vi>)
        n138 = call "setLabel.vi"("\"At\" location"=T4 {"XcoordSys"="graph", "YcoordSys"="graph", "Xvalue"=0.98, "Yvalue"=0.85} ("\"At\" location"), "Justify"="right", "multilineLabel"=w442, "String in"=w452) -> ("String out"=w451:string)  [unwired: 6 in, 1 out]
        n139 = call "getAxisBounds.vi"("Active Y Scale"=w462, "Active X Scale"=w462, "XYGraph in"=w465) -> ("Ybounds"=w463:T10, "Xbounds"=w464:T10)  [unwired: 5 in, 2 out]
        n140 = call "AssembleBLMultiplotScript-Spectra.vi"("gnuplotIn"=w451, "SpectrumFilename"=w460, "f.E(f) Bounds"=w463, "f Bounds"=w464) -> ("gnuplotOut"=w461:string)  [unwired: 11 in]
      }
      frame "Write gnuplot file" {
        w487 = FALSE  # append to file? (new file:F)
        w488 = FALSE  # advisory dialog? (display:T)
        n141 = call "chainCommands.vi"("Command"="unset multiplot\t", "Comments"="Close out multiplot", "StringIn"=w475) -> ("StringOut"=w474:string)  [unwired: 8 in]
        n142 = Build Path(base path=w480, name or relative path="gnuplot_script.txt") -> (appended path=w489:path)
        n143 = call "Write_Characters_To_File.vi"("file path (dialog if empty)"=w489, "advisory dialog? (display:T)"=w488, "character string"=w474, "append to file? (new file:F)"=w487) -> ()  [unwired: 1 in, 4 out]
      }
      frame "Execute shell script" {
        n144 = local read "Final Title"() -> (w494:string)
        n145 = Search and Replace String(replace all?=TRUE ("replace all? (F)"), input string=w494, search string=" ", replace string="\\ " ("replace string (\"\")")) -> (result string=w493:string)  [unwired: 4 in, 3 out]
        n146 = Build Path(base path=w496, name or relative path=w493) -> (appended path=w495:path)
        n147 = local read "OutputType"() -> (w491:enum16{"PDF", "PNG-ReportStyle"})
        n148 = call "Run_Gnuplot_Script.vi"("OutputType"=w491, "logfileName"=w504, "workingDirectory"=w495) -> ()
      }
      frame "Has pdf been generated?" {
        n149 = Select(t="Open Standard output file" ("f"), s="OpenLogfile?", f="UI-Monitor" ("t")) -> (s? t:f=w518:string)
        n150 = Select(t="Show Re-Run Gnuplot?", s="Show Script Editor?", f=w518) -> (s? t:f=w521:string)
        n151 = local read "autoprint"() -> (w511:bool)
        n152 = Not(x=w511) -> (.not. x?=w512:bool)
      }
      frame "Show Re-Run Gnuplot?" {
        n153 = local read "OutputType"() -> (w528:enum16{"PDF", "PNG-ReportStyle"})
        n154 = call "Re_run_Gnuplot.vi"("Plot folder (dialog if empty)"=w533, "OutputType"=w528) -> ()  [unwired: 3 out]
      }
      frame "Open Standard output file" {
        n155 = Format Into String(format string="open \"%s\"", w547) -> (resulting string=w546:string)  [unwired: 2 in, 1 out]
        n156 = call <vilib>:"System Exec.vi"("working directory"=w543, "command line"=w546) -> ()  [unwired: 4 in, 6 out]
      }
    }
    "case" <- w24
    "gnuplotScript" <- w21
    "File Path Control" <- w9
  }
  "Saved Automatically?" <- FALSE
